vi "TestExec.SN Valid and Route Check.vi"(6 "Process Steps":string[](array[string]), 7 "SN Indicator":refnum<vi>, 8 "ParamName":string="@SN", 9 "SN":string, 10 "Route Check":bool) -> (1 "Message":string, 2 "Status":bool, 4 "error IO":errorcluster, 5 "Inbound Process Step":string)   [LabVIEW 2018]
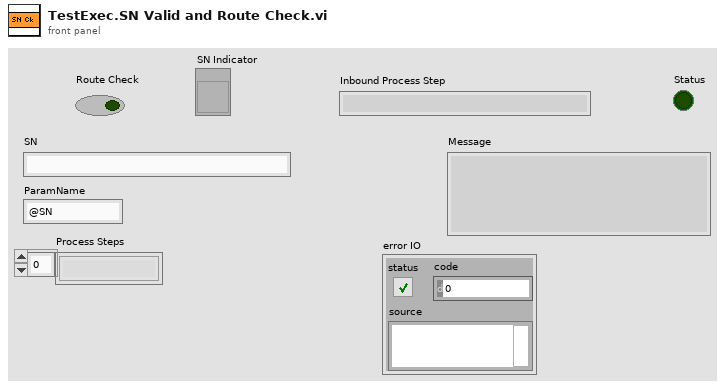
[diagram p1: front panel]
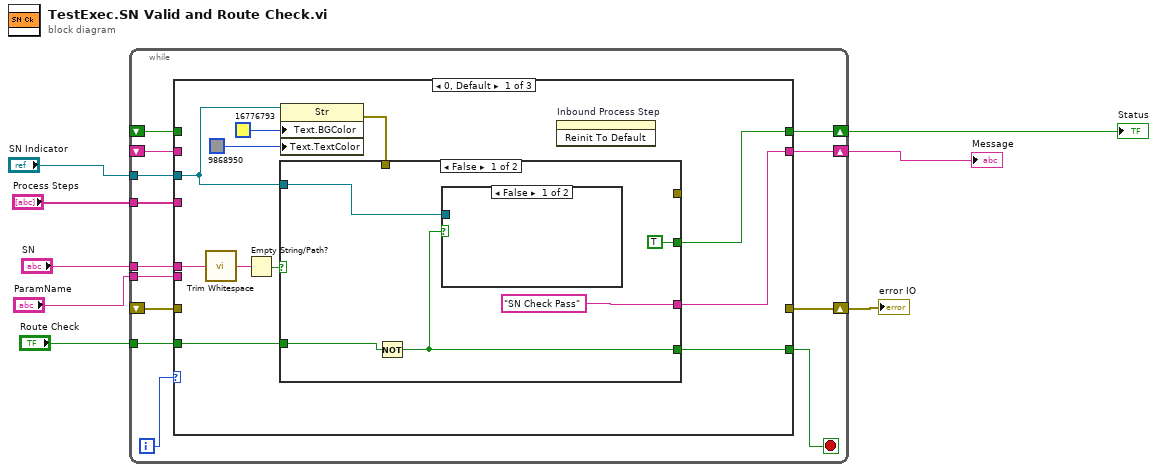
[diagram p0: block diagram]
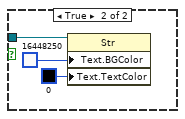
[diagram p2: hidden frame]
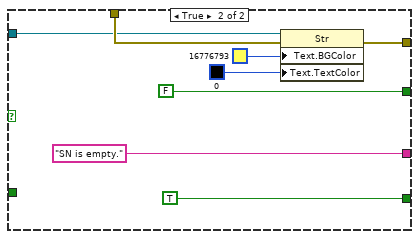
[diagram p3: hidden frame]
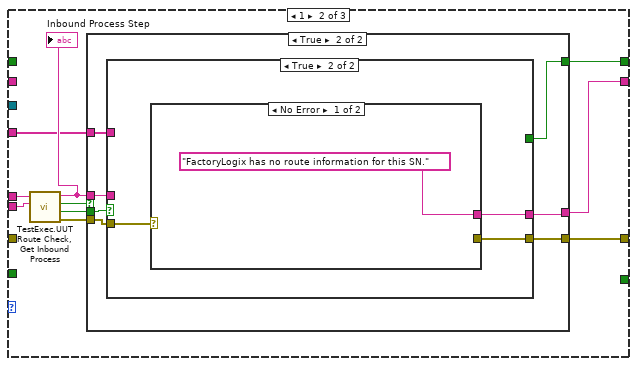
[diagram p4: hidden frame]
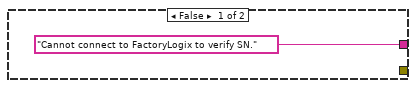
[diagram p5: hidden frame]
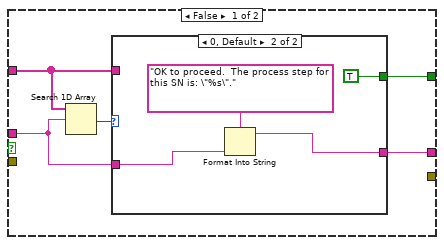
[diagram p6: hidden frame]
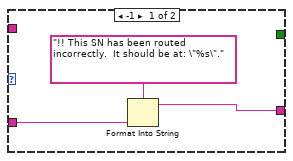
[diagram p7: hidden frame]
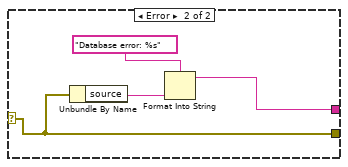
[diagram p8: hidden frame]
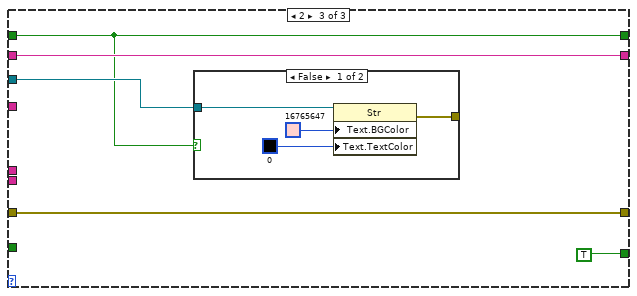
[diagram p9: hidden frame]
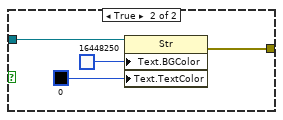
[diagram p10: hidden frame]
diagram:
  n1 = while {
    shift-right: [w16] -> w3
    shift-left: _ -> [w18]
    shift-right: [w15] -> w8
    shift-left: _ -> [w17]
    tunnel: "SN" -> [w20]
    tunnel: "Route Check" -> [w19]
    tunnel: "Process Steps" -> [w13]
    tunnel: "SN Indicator" -> [w12]
    shift-right: [w11] -> w2
    shift-left: _ -> [w10]
    tunnel: "ParamName" -> [w9]
    i -> [w21]
    stop <- w14 stop-if-true
    n2 = case shown="0, Default" w21 {
      tunnel: w20 -> [w31 w58 _]
      tunnel: w19 -> [w26 _ _]
      tunnel: w18 -> [_ _ w87]
      tunnel: w17 -> [_ _ w89]
      tunnel: [w29 w51 w87] -> w16
      tunnel: [w28 w55 w89] -> w15
      tunnel: [w27 _ TRUE] -> w14
      tunnel: w13 -> [_ w52 _]
      tunnel: w12 -> [w22 _ w88]
      tunnel: [_ w50 w91] -> w11
      tunnel: w10 -> [_ _ w91]
      tunnel: w9 -> [_ w49 _]
      frame 0, Default {
        n3 = call <vilib>:"Trim Whitespace.vi"("string"=w31) -> ("trimmed string"=w32:string)  [unwired: 1 in]
        n4 = Empty String/Path?(string/path=w32) -> (empty?=w30:bool)
        n5 = property class="Str"(reference=w22, "Text.BGColor"=u32 16776793, "Text.TextColor"=u32 9868950) -> (error out=w23:errorcluster)  [unwired: 1 in, 1 out]
        n6 = case shown="False" w30 {
          tunnel: [TRUE FALSE] -> w29
          tunnel: ["SN Check Pass" "SN is empty."] -> w28
          tunnel: [w33 TRUE] -> w27
          tunnel: w26 -> [w35 _]
          tunnel: w23 -> [_ w43]
          tunnel: [_ w42] -> _
          tunnel: w22 -> [w34 w41]
          frame False {
            n7 = Not(x=w35) -> (.not. x?=w33:bool)
            n8 = case shown="False" w33 {
              tunnel: w34 -> [_ w38]
              frame False {
              }
              frame True {
                n9 = property class="Str"(reference=w38, "Text.BGColor"=u32 16448250, "Text.TextColor"=u32 0) -> ()  [unwired: 1 in, 2 out]
              }
            }
          }
          frame True {
            n10 = property class="Str"(reference=w41, error in=w43, "Text.BGColor"=u32 16776793, "Text.TextColor"=u32 0) -> (error out=w42:errorcluster)  [unwired: 1 out]
          }
        }
        n11 = invoke on="Inbound Process Step" class="Str" method="Reinit To Default"() -> ()  [unwired: 3 in, 3 out]
      }
      frame 1 {
        n12 = call "TestExec.UUT Route Check, Get Inbound Process.vi"("parameter name"=w49, "UUT SN"=w58) -> ("error out"=w56:errorcluster, "No Data"=w53:bool, "Connected"=w57:bool, "Inbound Process Step"=w54:string)  [unwired: 6 in]
        "Inbound Process Step" <- w54
        n13 = case shown="True" w57 {
          tunnel: w56 -> [_ w61]
          tunnel: ["Cannot connect to FactoryLogix to verify SN." w64] -> w55
          tunnel: w54 -> [_ w65]
          tunnel: w53 -> [_ w66]
          tunnel: w52 -> [_ w63]
          tunnel: [_ w62] -> w51
          tunnel: [_ w60] -> w50
          frame False {
          }
          frame True {
            n14 = case shown="True" w66 {
              tunnel: w65 -> [w69 _]
              tunnel: [w68 w81] -> w64
              tunnel: w63 -> [w71 _]
              tunnel: [w67 _] -> w62
              tunnel: w61 -> [_ w80]
              tunnel: [_ w79] -> w60
              frame False {
                n15 = Search 1D Array(1D array=w71, element=w69) -> (index of element=w70:i32)  [unwired: 1 in]
                n16 = case shown="0, Default" w70 {
                  tunnel: w71 -> [_ _]
                  tunnel: w69 -> [w73 w75]
                  tunnel: [w72 w76] -> w68
                  tunnel: [_ TRUE] -> w67
                  frame -1 {
                    n17 = Format Into String(format string="!! This SN has been routed incorrectly.  It should be at: \"%s\".", w73) -> (resulting string=w72:string)  [unwired: 2 in, 1 out]
                  }
                  frame 0, Default {
                    n18 = Format Into String(format string="OK to proceed.  The process step for this SN is: \"%s\".", w75) -> (resulting string=w76:string)  [unwired: 2 in, 1 out]
                  }
                }
              }
              frame True {
                n19 = case shown="No Error" w80 {
                  selector: w80 -> [_ w84]
                  tunnel: ["FactoryLogix has no route information for this SN." w85] -> w81
                  tunnel: [_ w84] -> w79
                  frame No Error {
                  }
                  frame Error {
                    n20 = Unbundle By Name(w84) -> ("source"=w83:string)
                    n21 = Format Into String(format string="Database error: %s", w83) -> (resulting string=w85:string)  [unwired: 2 in, 1 out]
                  }
                }
              }
            }
          }
        }
      }
      frame 2 {
        n22 = case shown="False" w87 {
          tunnel: w88 -> [w94 w97]
          tunnel: [w93 w96] -> _
          frame False {
            n23 = property class="Str"(reference=w94, "Text.BGColor"=u32 16765647, "Text.TextColor"=u32 0) -> (error out=w93:errorcluster)  [unwired: 1 in, 1 out]
          }
          frame True {
            n24 = property class="Str"(reference=w97, "Text.BGColor"=u32 16448250, "Text.TextColor"=u32 0) -> (error out=w96:errorcluster)  [unwired: 1 in, 1 out]
          }
        }
      }
    }
  }
  "Message" <- w8
  "Status" <- w3
  "error IO" <- w2
